vi "lvpeak_load_config.vi"(8 "error in (no error)":errorcluster, 10 "config path":path, 11 "camera_id":u64) -> (0 "error out":errorcluster, 3 "camera_id out":u64)   [LabVIEW 2024, in "Vision.lvlib"]
uses:
  Vision.lvlib
  bin/LVPeak.dll
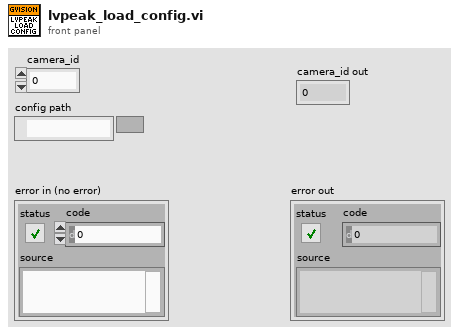
[diagram p1: front panel]
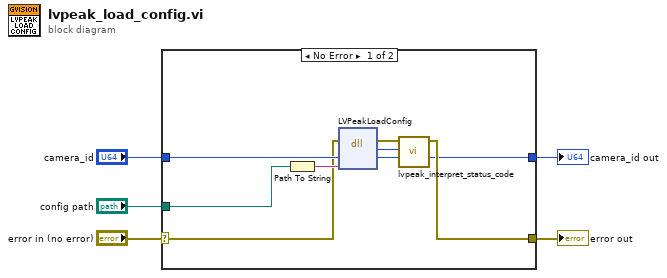
[diagram p0: block diagram]
diagram:
  n1 = case shown="No Error" "error in (no error)" {
    selector: "error in (no error)" -> [w10 w15]
    tunnel: "camera_id" -> [w13 w14]
    tunnel: [w7 w15] -> w3
    tunnel: "config path" -> [w12 _]
    tunnel: [w6 w14] -> w1
    frame No Error {
      n2 = Path To String(path=w12) -> (string=w11:string)
      n3 = dll-call lib="C:/Users/cfang/Desktop/nebraska-silicon-lab/pixel-gantry-control/Gantry/Shared Components/bin/LVPeak.dll" fn="LVPeakLoadConfig"(error in=w10, "camera_id"=w13, "filename"=w11) -> (error out=w9:errorcluster, "return type"=w8:i32, "camera_id"=w6:u64)  [unwired: 3 in, 1 out]
      n4 = call "lvpeak_interpret_status_code.vi"("status_code"=w8, "error in (no error)"=w9) -> ("error out"=w7:errorcluster)  [unwired: 9 in]
    }
    frame Error {
    }
  }
  "error out" <- w3
  "camera_id out" <- w1
